vi "ABB Sort 2D Array.vi"(4 "Column/Row to Sort By":u32, 6 "Unsorted 2D Array":dbl[][](array[numeric])=[[0.0, 0.0, 0.0], [0.0, 0.0, 0.0], [0.0, 0.0, 0.0], [0.0, 0.0, 0.0], [0.0, 0.0, 0.0], [0.0, 0.0, 0.0]] format="%.2f", 7 "Sort by":enum16{"Column", "Row"}(ring)) -> (2 "Sorted 2D Array":dbl[][](array[numeric]) format="%.2f")   [LabVIEW 2017]
doc: "This VI sorts a 2D array of any size in descending or ascending order\nbased on a column or row whose index you specify. It does not use\na secondary column/row to sort by, so, if the main column/row has\nmultiple elements that have the same value, the first of those elements\nthat is found in the original array is going to be the element placed first\nin the sorted array. To use, enter an array in the 2D Array and select\nwhether to sort by Ascending or Descending order and whether to sort\nbased on a column or row and the index of that column or row. This\nVI can also be used as a SubVI and the Values can be passed to it."
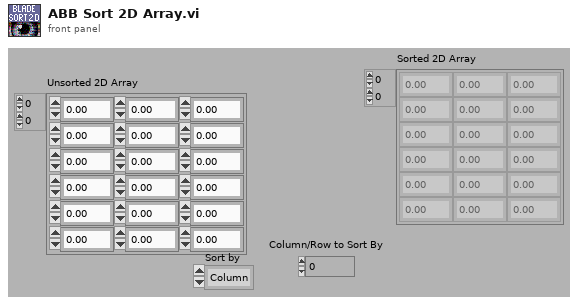
[diagram p1: front panel]
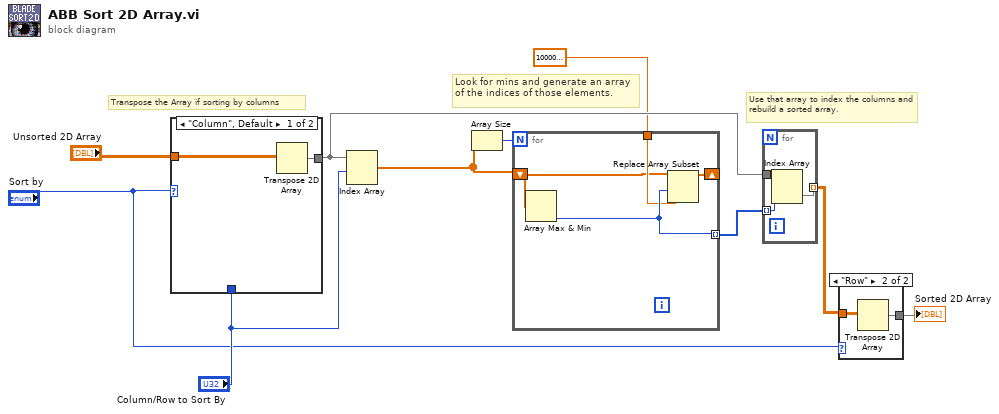
[diagram p0: block diagram]
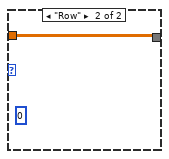
[diagram p3: hidden frame]
diagram:
  # "Use that array to index the columns and rebuild a sorted array."
  # "Look for mins and generate an array of the indices of those elements."
  # "Transpose the Array if sorting by columns"
  n1 = case shown="\"Column\", Default" "Sort by" {
    tunnel: "Unsorted 2D Array" -> [w12 w13]
    tunnel: [w11 w13] -> w9
    tunnel: "Column/Row to Sort By" -> [_ _]
    frame "Column", Default {
      n2 = Transpose 2D Array(2D array=w12) -> (transposed array=w11:dbl[][])
    }
    frame "Row" {
      (unwired) 0 ("Index")
    }
  }
  n3 = Index Array(array=w9, index (row)="Column/Row to Sort By") -> (element=w3:dbl[])  [unwired: 1 in]
  n4 = Array Size(array=w3) -> (size(s)=w10:i32)
  n5 = for {
    N: w10 -> [_]
    shift-right: [w17] -> _
    shift-left: w3 -> [w14]
    tunnel: [w16] -> w7 mode=indexing
    tunnel: 1000000000.0 -> [w15]
    n6 = Array Max & Min(array=w14) -> (min index (indices)=w16:i32)  [unwired: 3 out]
    n7 = Replace Array Subset(array=w14, new element=w15, index=w16) -> (w17:dbl[])
  }
  n8 = for {
    tunnel: w7 -> [w20] mode=indexing
    tunnel: w9 -> [w19]
    tunnel: [w18] -> w8 mode=indexing
    n9 = Index Array(array=w19, index (col)=w20) -> (element=w18:dbl[])  [unwired: 1 in]
  }
  n10 = case shown="\"Row\"" "Sort by" {
    tunnel: w8 -> [w21 w23]
    tunnel: [w21 w22] -> w6
    frame "Column", Default {
    }
    frame "Row" {
      n11 = Transpose 2D Array(2D array=w23) -> (transposed array=w22:dbl[][])
    }
  }
  "Sorted 2D Array" <- w6
